vi "Setup UI.vi"(8 "error in (no error)":errorcluster, 10 "Set UI to input? (F)":bool, 11 "Varian Continuous in":refnum<class "Varian Continuous.lvclass">) -> (0 "error out":errorcluster, 3 "Varian Continuous out":refnum<class "Varian Continuous.lvclass">)   [LabVIEW 2009, in "Varian Continuous.lvclass"]
doc: "Scanner::Setup is a constructor that has no parameters and faces the user. The Factory calls this VI to let the user configure this Scanner. It is dynamically dispatched in order to let the user choose the type as well as the options of the scanner."
uses:
  Varian Continuous.lvclass
  Scanner/Scanner.lvclass
  Varian Continuous.lvclass/Varian Continuous.ctl
  Instruments/Varian Magnet/Varian Magnet.lvclass
panel:
  out "Calibrating":bool
  in  "calibrate magnet":bool
  in  "Voltage Control":u16(ring) items=["Please Select a Value", "30V", "40V"]
  in  "Sweep Rate":dbl[unit]
  # "VOLTAGE KNOB SETTINGS:\n\nMAIN SETTING:\n40 V on High Voltage Knob\n\nFor fields 0.1 T increasing  0.45 T\n fast response and all decreasing fields\nP= -350\nI= -12\nD= 1\n\nFor fields 0.5 T increasing to 0.9 T\nuse PID gains with smallest peak and \nfastest response\nP= -75\nI= -0.5\nD= -1\n\nDO NOT GO ABOVE 0.9 T\n\n\n30 V SETTING:\nBest for fields below 0.5 T. 0.5 MAX comfortable range. Faster with fields below 0.1 T than on the 40 V setting.\nP= -110\nI= -2\nD= 1\n\n50 V SETTING:\nNot reliable"
  # "Varian Continuous Control"
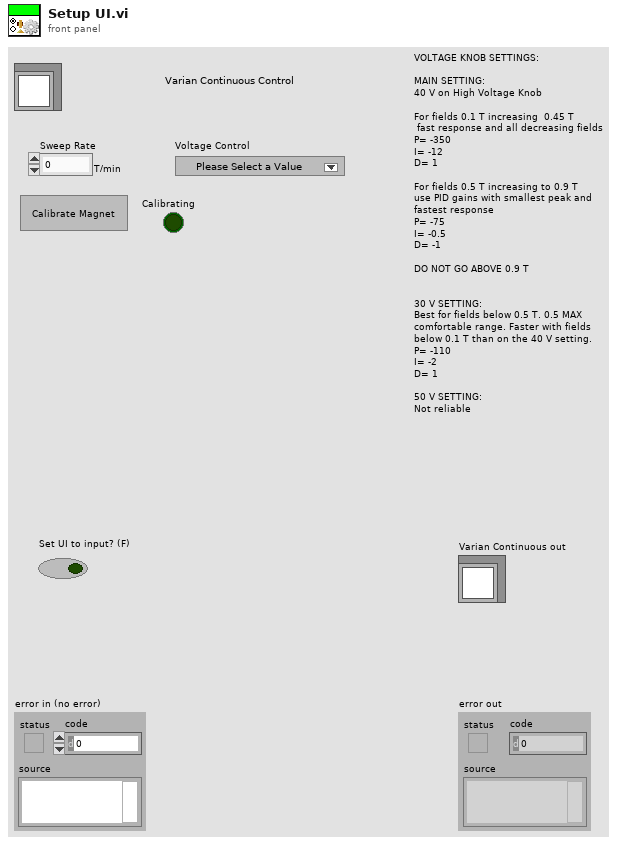
[diagram p1: front panel]
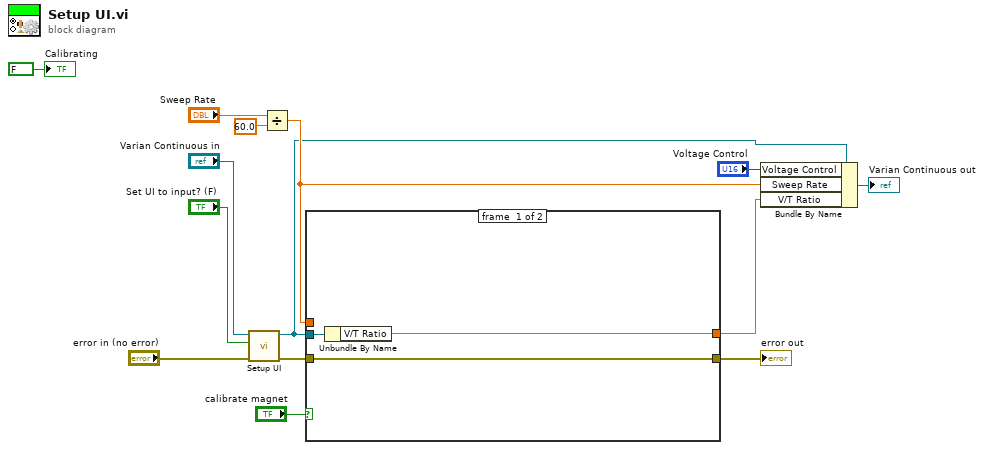
[diagram p0: block diagram]
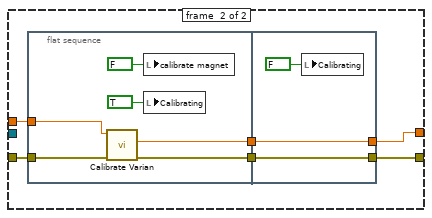
[diagram p2: hidden frame]
diagram:
  n1 = call-parent "Setup UI.vi"("error in (no error)"="error in (no error)", "Set UI to input? (F)"="Set UI to input? (F)", "Scanner in"="Varian Continuous in") -> ("error out"=w6:errorcluster, "Scanner out"=w3:refnum<class "Varian Continuous.lvclass">)  [unwired: 7 in]
  n2 = Divide(x="Sweep Rate", y=60.0) -> (x/y=w7:dbl[unit])
  n3 = case shown="True" "calibrate magnet" {
    tunnel: w7 -> [_ w23]
    tunnel: w6 -> [w17 w22]
    tunnel: [w17 w21] -> w5
    tunnel: [w15 w18] -> w4
    tunnel: w3 -> [w16 _]
    frame #0 {
      n4 = Unbundle By Name(w16) -> ("V/T Ratio"=w15:dbl[unit])
    }
    frame #1 {
      n5 = flat-sequence {
        tunnel: w23 -> [w28]
        tunnel: w22 -> [w27]
        tunnel: [w26] -> w20
        tunnel: [w25] -> w19
        tunnel: [w31] -> w18
        tunnel: [w32] -> w21
        tunnel: w20 -> [w32]
        tunnel: w19 -> [w31]
        frame #0 {
          n6 = call "Calibrate Varian.vi"("error in"=w27, "Sweep Rate"=w28) -> ("error out"=w26:errorcluster, "V/T ratio"=w25:dbl[unit])  [unwired: 8 in]
          n7 = local write "calibrate magnet"(FALSE ("calibrate magnet")) -> ()
          n8 = local write "Calibrating"(TRUE ("Calibrating")) -> ()
        }
        frame #1 {
          n9 = local write "Calibrating"(FALSE ("calibrate magnet")) -> ()
        }
      }
    }
  }
  "error out" <- w5
  n10 = Bundle By Name(cluster=w3, "Voltage Control"="Voltage Control", "Sweep Rate"=w7, "V/T Ratio"=w4) -> (→"Varian Continuous out":refnum<class "Varian Continuous.lvclass">)
  "Calibrating" <- FALSE ("Calibrating")
